vi "dateacq.vi"(11 "date format (0)":enum16{"short", "long", "abbreviated"}(ring)) -> (0 "Month":i32, 1 "time string":string, 2 "substring before match":string, 3 "date string":string)   [LabVIEW 2013]
panel:
  out "substring":string
  out "match + rest of string":string
  # "Year of Study Analysis"
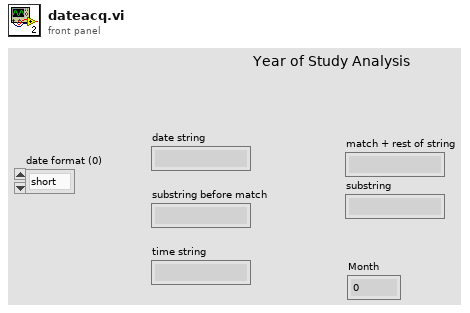
[diagram p1: front panel]
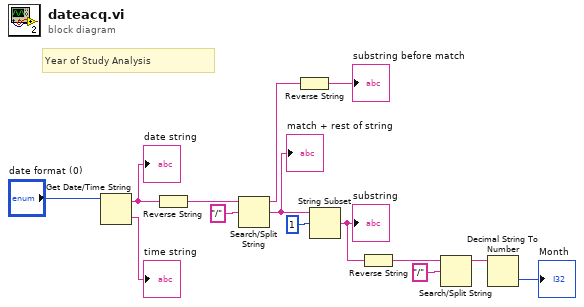
[diagram p0: block diagram]
diagram:
  # "Year of Study Analysis"
  n1 = Get Date/Time String(date format (0)="date format (0)") -> (date string=w11:string, time string=→"time string":string)  [unwired: 2 in]
  "date string" <- w11
  n2 = Reverse String(1:w11) -> (0:w12:string)
  n3 = Search/Split String(string=w12, search string/char (-)="/") -> (substring before match=w13:string, match + rest of string=w7:string)  [unwired: 1 in, 1 out]
  "match + rest of string" <- w7
  n4 = Reverse String(1:w13) -> (0:→"substring before match":string)
  n5 = String Subset(string=w7, offset (0)=1) -> (substring=w5:string)  [unwired: 1 in]
  "substring" <- w5
  n6 = Reverse String(1:w5) -> (0:w4:string)
  n7 = Search/Split String(string=w4, search string/char (-)="/") -> (substring before match=w2:string)  [unwired: 1 in, 2 out]
  n8 = Decimal String To Number(string=w2) -> (number=→"Month":i32)  [unwired: 2 in, 1 out]
